vi "save_settings.vi"(8 "error in":errorcluster) -> (0 "error out":errorcluster, 3 "XML String":string)   [LabVIEW 2011]
uses:
  Functional Globals/Pulse Parameters.ctl
  Functional Globals/Hardware Parameters.ctl
  <vilib>/Utility/xml.llb/Write to XML File(string).vi
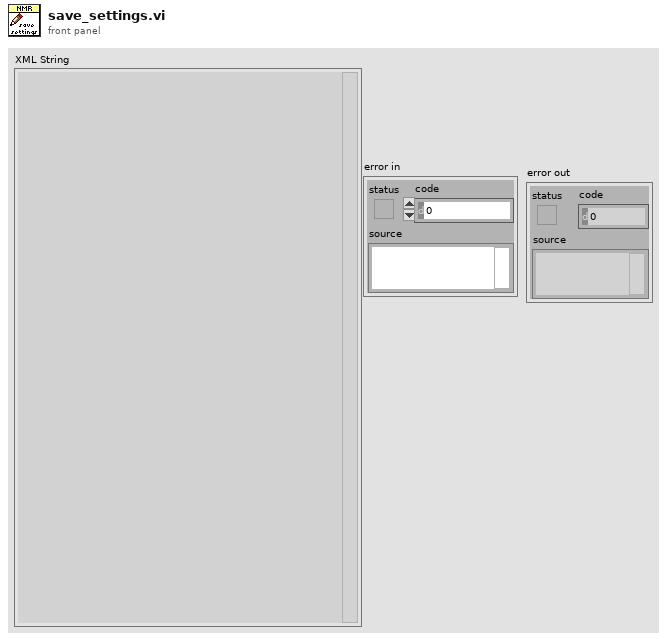
[diagram p1: front panel]
types:
  T1 = typedef "Hardware Parameters.ctl" = enum16{"Initialize", "Set Hardware Settings", "Get Hardware Settings", "Get Hardware CMD String"}
  T2 = typedef "Pulse Parameters.ctl" = enum16{"Initialize", "Set T1 Pulse Settings", "Set 90 Degree Pulse Settings", "Set CPMG Pulse Settings", "Get T1 Settings", "Get CPMG Settings", "Get 90 Degree Settings"}
  T3 = typedef "90D_Delay Settings.ctl" = cluster{"Delay d1":dbl, "Delay d2":dbl, "d1 Unit":u8, "d2 Unit":u8}
  T4 = typedef "90D_Preliminary Settings.ctl" = cluster{"Nº of Scans (ns)":u16, "Pulse Frequency":dbl}
  T5 = typedef "90D_Pulse Settings.ctl" = cluster{"Duration Signal P1":dbl, "Power Level":u16, "Phase":u16, "P1 Units":u8}
  T6 = typedef "Acquisition Settings.ctl" = cluster{"Number Samples":u16, "Time Between Points":dbl, "Unit":u8}
  T7 = cluster{"Delay Settings":T3, "Preliminary Settings":T4, "Pulse Settings":T5, "Acquisition Settings":T6}
  T8 = typedef "CPMG_Delay Settings.ctl" = cluster{"Delay d1":dbl, "Delay d2":dbl, "d1 Unit":u8, "d2 Unit":u8, "Delay d3":dbl, "d3 Unit":u8, "Delay d4":dbl, "d4 Unit":u8}
  T9 = typedef "CPMG_Preliminary Settings.ctl" = cluster{"Nº of Scans (ns)":u16, "Pulse Frequency":dbl, "Nº of Echoes (ne)":u16}
  T10 = typedef "CPMG_Pulse Settings.ctl" = cluster{"Duration Signal P1":dbl, "Power Level P1":u16, "Phase P1":u16, "P1 Unit":u8, "Duration Signal P2":dbl, "Power Level P2":u16, "Phase P2":u16, "P2 Unit":u8}
  T11 = cluster{"Acquisition Settings":T6, "Delay Settings":T8, "Preliminary Settings":T9, "Pulse Settings":T10}
  T12 = typedef "T1_Preliminary Settings.ctl" = cluster{"Nº of Scans (ns)":u16, "Pulse Frequency":dbl, "Nº of Vd":u16}
  T13 = typedef "T1_Pulse Settings.ctl" = cluster{"Duration Signal P2":dbl, "Power Level P2":u16, "Phase P2":u16, "P2 Unit":u8, "Duration Signal P1":dbl, "Power Level P1":u16, "Phase P1":u16, "P1 Unit":u8}
  T14 = typedef "T1_Delay Settings.ctl" = cluster{"Delay d1":dbl, "Delay d2":dbl, "d1 Unit":u8, "d2 Unit":u8, "Delay d30":dbl, "d30 Unit":u8, "Vd Unit":u8, "Vd Values":string}
  T15 = cluster{"Preliminary Settings":T12, "Pulse Settings":T13, "Acquisition Settings":T6, "Delay Settings":T14}
  T16 = typedef "Hardware Control.ctl" = cluster{"Number Samples":u16, "Time Between Points":dbl, "Gain2 (dB)":i8, "CuttOff Freq1[MHz]":u8, "CuttOff Freq2[MHz]":u8, "Frequency":dbl, "Phase":u16, "Power Level":u16, "Send Pulse":bool, "Reset DDS":bool, "TX CTRL":bool, "RX CTRL":bool, "Gain1 (dB)":i8, "Set DDS":bool, "Start AQS":bool, "Units":u8}
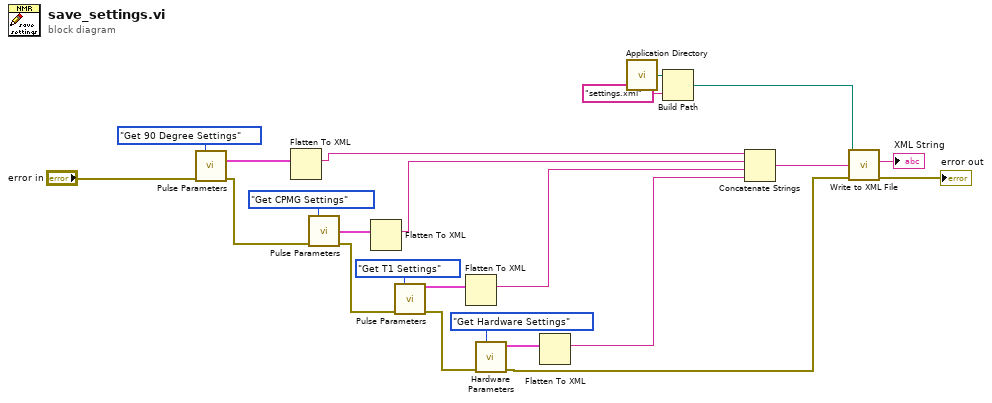
[diagram p0: block diagram]
diagram:
  n1 = call "Pulse Parameters.vi"("action"=Pulse_Parameters."Get 90 Degree Settings", "error in"="error in") -> ("90 Degree Pulse settings out"=w18:T7, "error out"=w12:errorcluster)  [unwired: 6 in, 6 out]
  n2 = Flatten To XML(anything=w18) -> (xml string=w23:string)
  n3 = call "Pulse Parameters.vi"("action"=Pulse_Parameters."Get CPMG Settings", "error in"=w12) -> ("CPMG pulse settings Out"=w14:T11, "error out"=w11:errorcluster)  [unwired: 6 in, 6 out]
  n4 = Flatten To XML(anything=w14) -> (xml string=w22:string)
  n5 = call "Pulse Parameters.vi"("action"=Pulse_Parameters."Get T1 Settings", "error in"=w11) -> ("T1 Pulse settings Out"=w15:T15, "error out"=w9:errorcluster)  [unwired: 6 in, 6 out]
  n6 = Flatten To XML(anything=w15) -> (xml string=w21:string)
  n7 = call "Hardware Parameters.vi"("action"=Hardware_Parameters."Get Hardware Settings", "error in"=w9) -> ("error out"=w10:errorcluster, "Hardware Paramentes out"=w7:T16)  [unwired: 8 in]
  n8 = Flatten To XML(anything=w7) -> (xml string=w6:string)
  n9 = call <vilib>:"Application Directory.vi"() -> ("Application Directory"=w3:path)
  n10 = Build Path(base path=w3, name or relative path="settings.xml") -> (appended path=w2:path)
  n11 = Concatenate Strings(w23, w22, w21, w6) -> (w20:string)
  n12 = call-poly <vilib>:"Write to XML File.vi"("error in (no error)"=w10, "XML Input"=w20, "XML File Path"=w2) -> ("error out"=→"error out":errorcluster, "XML String"=→"XML String":string)  [unwired: 2 in, 5 out]
